vi "Node Extract Message.vi"(6 "Paras In":variant, 8 "error in (no error)":errorcluster, 9 "Priority":i32, 10 "Wait":i32=-1, 11 "Node Actor in":refnum<class "Node Actor.lvclass">) -> (0 "error out":errorcluster, 1 "Valid":bool, 2 "Message Out":refnum<class "Message.lvclass">, 3 "Node Actor out":refnum<class "Node Actor.lvclass">)   [LabVIEW 2024, in "Node Actor.lvclass"]
uses:
  Node Actor.lvclass
  C:/Users/iio/Desktop/Bussiness/Tricorn Re/Madelbrot 4.0/General Library/Ancestor Class/Actor/System Actor/System Actor.lvclass
  Message/Message.lvclass
  System Actor/System Actor.lvclass/System Actor.ctl
  Node Actor.lvclass/Node Actor.ctl
  Messenger/Messenger/Messenger.lvclass
  9852db37-bd21-45e2-a4bb-d13c558760c8.vi
  System Actor/Public Data/Read Self Messenger Location.vi
  Messenger/Mail Strategy/Mail Strategy.lvclass
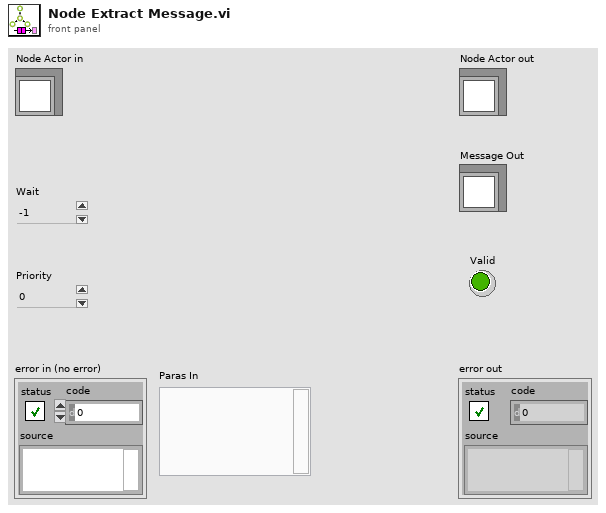
[diagram p1: front panel]
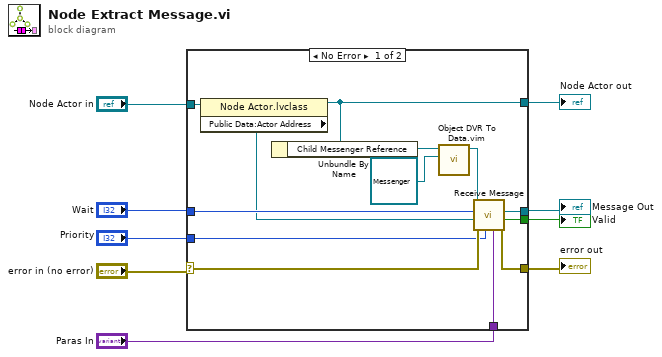
[diagram p0: block diagram]
diagram:
  n1 = case shown="No Error" "error in (no error)" {
    selector: "error in (no error)" -> [w20 w24]
    tunnel: [w19 w24] -> w3
    tunnel: [w13 w23] -> w8
    tunnel: "Node Actor in" -> [w17 w23]
    tunnel: [w22 _] -> w1
    tunnel: [w21 _] -> w2
    tunnel: "Wait" -> [w18 _]
    tunnel: "Priority" -> [w16 _]
    tunnel: "Paras In" -> [w15 _]
    frame No Error {
      n2 = property class="Node Actor.lvclass"(reference=w17) -> (reference out=w13:refnum<class "Node Actor.lvclass">, "Public Data:Actor Address"=w14:refnum<class "Mail Strategy.lvclass">)  [unwired: 1 in, 1 out]
      n3 = Unbundle By Name(w13) -> ("Child Messenger Reference"=w12:refnum<data-value>)
      n4 = call "Object DVR To Data.vim"("Class Type"=refnum<class "Messenger.lvclass"> refnum ("Public Data:Messenger"), "Object DVR In"=w12) -> ("Object Out"=w10:refnum<class "Messenger.lvclass">)  [unwired: 8 in, 1 out]
      n5 = call-dynamic "Receive Message.vi"("Paras In"=w15, "Priority"=w16, "error in (no error)"=w20, "Mail Strategy In"=w14, "Wait(ms)"=w18, "Messenger Component in"=w10) -> ("error out"=w19:errorcluster, "Valid"=w21:bool, "Message Out"=w22:refnum<class "Message.lvclass">)  [unwired: 2 in, 1 out]
    }
    frame Error {
    }
  }
  "error out" <- w3
  "Node Actor out" <- w8
  "Message Out" <- w1
  "Valid" <- w2
